vi "Load saved scan settings_arbitray cluster elements.vi"(8 "error in (no error)":errorcluster, 11 "User name":string) -> (0 "error out":errorcluster, 1 "Scan settings array":T1[](array[typedef]) {"J-t Illumination conditions" items=["Light only", "Dark only", "Light then dark", "Dark then light"]; "No. of scan rate steps" min=1.0 step=1.0; "Illumination conditions" items=["Light only", "Dark only", "Light then dark", "Dark then light", "Light then dark then light", "Dark then light then dark"]; "Time Constant (s)" items=["0.003", "0.01", "0.03", "0.1", "0.3", "1", "3", "10", "30", "100"]; "Only repeat for best pixel" items=["only for best pixel", "for best 2 pixels", "for best 3 pixels", "for best 4 pixels", "for best 5 pixels", "for best 6 pixels", "for best 7 pixels", "for all pixels"]; "No. of repeat scans" min=1.0 step=1.0; "EQE best pixel only" items=["only the best pixel", "the best 2 pixel", "the best 3 pixel", "the best 4 pixel", "the best 5 pixel", "the best 6 pixel", "the best 7 pixel", "all pixels"]; "P dep best pixel only" items=["only the best pixel", "the best 2 pixels", "the best 3 pixels", "the best 4 pixels", "the best 5 pixels", "the best 6 pixels", "the best 7 pixels", "all pixels"]; "Max power best pixel only" items=["only the best pixel", "the best 2 pixels", "the best 3 pixels", "the best 4 pixels", "the best 5 pixels", "the best 6 pixels", "the best 7 pixels", "all pixels"]; "J-t best pixel only" items=["only the best pixel", "the best 2 pixels", "the best 3 pixels", "the best 4 pixels", "the best 5 pixels", "the best 6 pixels", "the best 7 pixels", "all pixels"]; "Integration time" items=["Fast", "Normal", "High Accuracy"]; "Stabilisation mode" items=["V", "I"]; "Measurement delay (ms)" min=10.0}, 3 "Scan settings name array":string[](array[string]), 4 "Settings folder path":path)   [LabVIEW 2011]
uses:
  TypeDefs/Scan settings.ctl
  TypeDefs/Settings Boolean.ctl
  <vilib>/Utility/file.llb/Write To Spreadsheet File (string).vi
  <vilib>/Utility/file.llb/Read From Spreadsheet File (string).vi
panel:
  in  "Deafult_std":string[](array[string])=["1", "0", "-1.4", "0.1", "0.02", "10", "1", "0", "5", "0", "-1.4", "0", "0", "0", "0", "1", "1", "0", "0", "1", "0", "1", "0.7", "60", "0", "7", "0", "0", "0", "0", "0", "300", "900", "5", "100", "2", "3", "90", "2", "1", "2", "1", "1", "1", "0", "1", "0", "200", "0"]
  in  "Deafult_inv":string[](array[string])=["1", "0", "-0.1", "1.4", "0.02", "10", "1", "1", "0", "0", "1.4", "0", "0", "0", "0", "1", "1", "0", "0", "1", "0", "1", "0.7", "60", "0", "7", "0", "0", "0", "0", "0", "300", "900", "5", "100", "2", "3", "90", "2", "1", "2", "1", "1", "1", "0", "1", "0", "200", "0"]
  out "String":string
  out "all rows":string[][](array[string])
  in  "Scan settings":T1={"J-V scan"=TRUE, "J-t scan"=FALSE, "Min voltage (V)"=0.0, "Max voltage (V)"=1.4, "Step (V)"=0.01, "Measurement delay (ms)"=10.0, "1st scan FB-SC"=TRUE, "Inverted structure"=FALSE, "Stabilisation time (s)"=0.0, "Stabilisation mode"=0, "Stabilisation value (V or A) "=0.0, "Step time (s)"=1.0, "Integration time"=0, "Repeat light scans"=FALSE, "Stabilisation in the dark?"=FALSE, "J-t Min (V)"=0.0, "J-t Max (V)"=1.4, "J-t Step (V)"=0.01, "Max. power stabilisation"=FALSE, "J-t 1st scan FB-SC"=TRUE, "J-t Inverted structure"=FALSE, "Max power tracking"=FALSE, "Vmp (V)"=0.7, "Total stabilisation time (s)"=100.0, "J-t best pixel only"=0, "Max power best pixel only"=0, "Vmp from J-V scan"=FALSE, "Intensity dependence"=FALSE, "P dep best pixel only"=0, "External quantum efficiency"=FALSE, "EQE best pixel only"=0, "WL min (nm)"=300.0, "WL max (nm)"=900.0, "WL step (nm)"=5.0, "Wait (ms)"=100.0, "No. of repeat scans"=2.0, "Only repeat for best pixel"=0, "Chopper Freq.  (Hz)"=90.0, "Time Constant (s)"=2.0, "Stabilisation time step (s)"=1.0, "Illumination conditions"=2, "Scan rate min (V/s)"=0.1, "Scan rate max (V/s)"=1.0, "No. of scan rate steps"=1.0, "Scan rate voltage step priority"=FALSE, "Scan rate measurement delay priority"=FALSE, "J-t Illumination conditions"=0, "White bias  (no. of suns)"=200.0, "Max P stab. Specific voltage"=FALSE} {"J-t Illumination conditions" items=["Light only", "Dark only", "Light then dark", "Dark then light"]; "No. of scan rate steps" min=1.0 step=1.0; "Illumination conditions" items=["Light only", "Dark only", "Light then dark", "Dark then light", "Light then dark then light", "Dark then light then dark"]; "Time Constant (s)" items=["0.003", "0.01", "0.03", "0.1", "0.3", "1", "3", "10", "30", "100"]; "Only repeat for best pixel" items=["only for best pixel", "for best 2 pixels", "for best 3 pixels", "for best 4 pixels", "for best 5 pixels", "for best 6 pixels", "for best 7 pixels", "for all pixels"]; "No. of repeat scans" min=1.0 step=1.0; "EQE best pixel only" items=["only the best pixel", "the best 2 pixel", "the best 3 pixel", "the best 4 pixel", "the best 5 pixel", "the best 6 pixel", "the best 7 pixel", "all pixels"]; "P dep best pixel only" items=["only the best pixel", "the best 2 pixels", "the best 3 pixels", "the best 4 pixels", "the best 5 pixels", "the best 6 pixels", "the best 7 pixels", "all pixels"]; "Max power best pixel only" items=["only the best pixel", "the best 2 pixels", "the best 3 pixels", "the best 4 pixels", "the best 5 pixels", "the best 6 pixels", "the best 7 pixels", "all pixels"]; "J-t best pixel only" items=["only the best pixel", "the best 2 pixels", "the best 3 pixels", "the best 4 pixels", "the best 5 pixels", "the best 6 pixels", "the best 7 pixels", "all pixels"]; "Integration time" items=["Fast", "Normal", "High Accuracy"]; "Stabilisation mode" items=["V", "I"]; "Measurement delay (ms)" min=10.0}
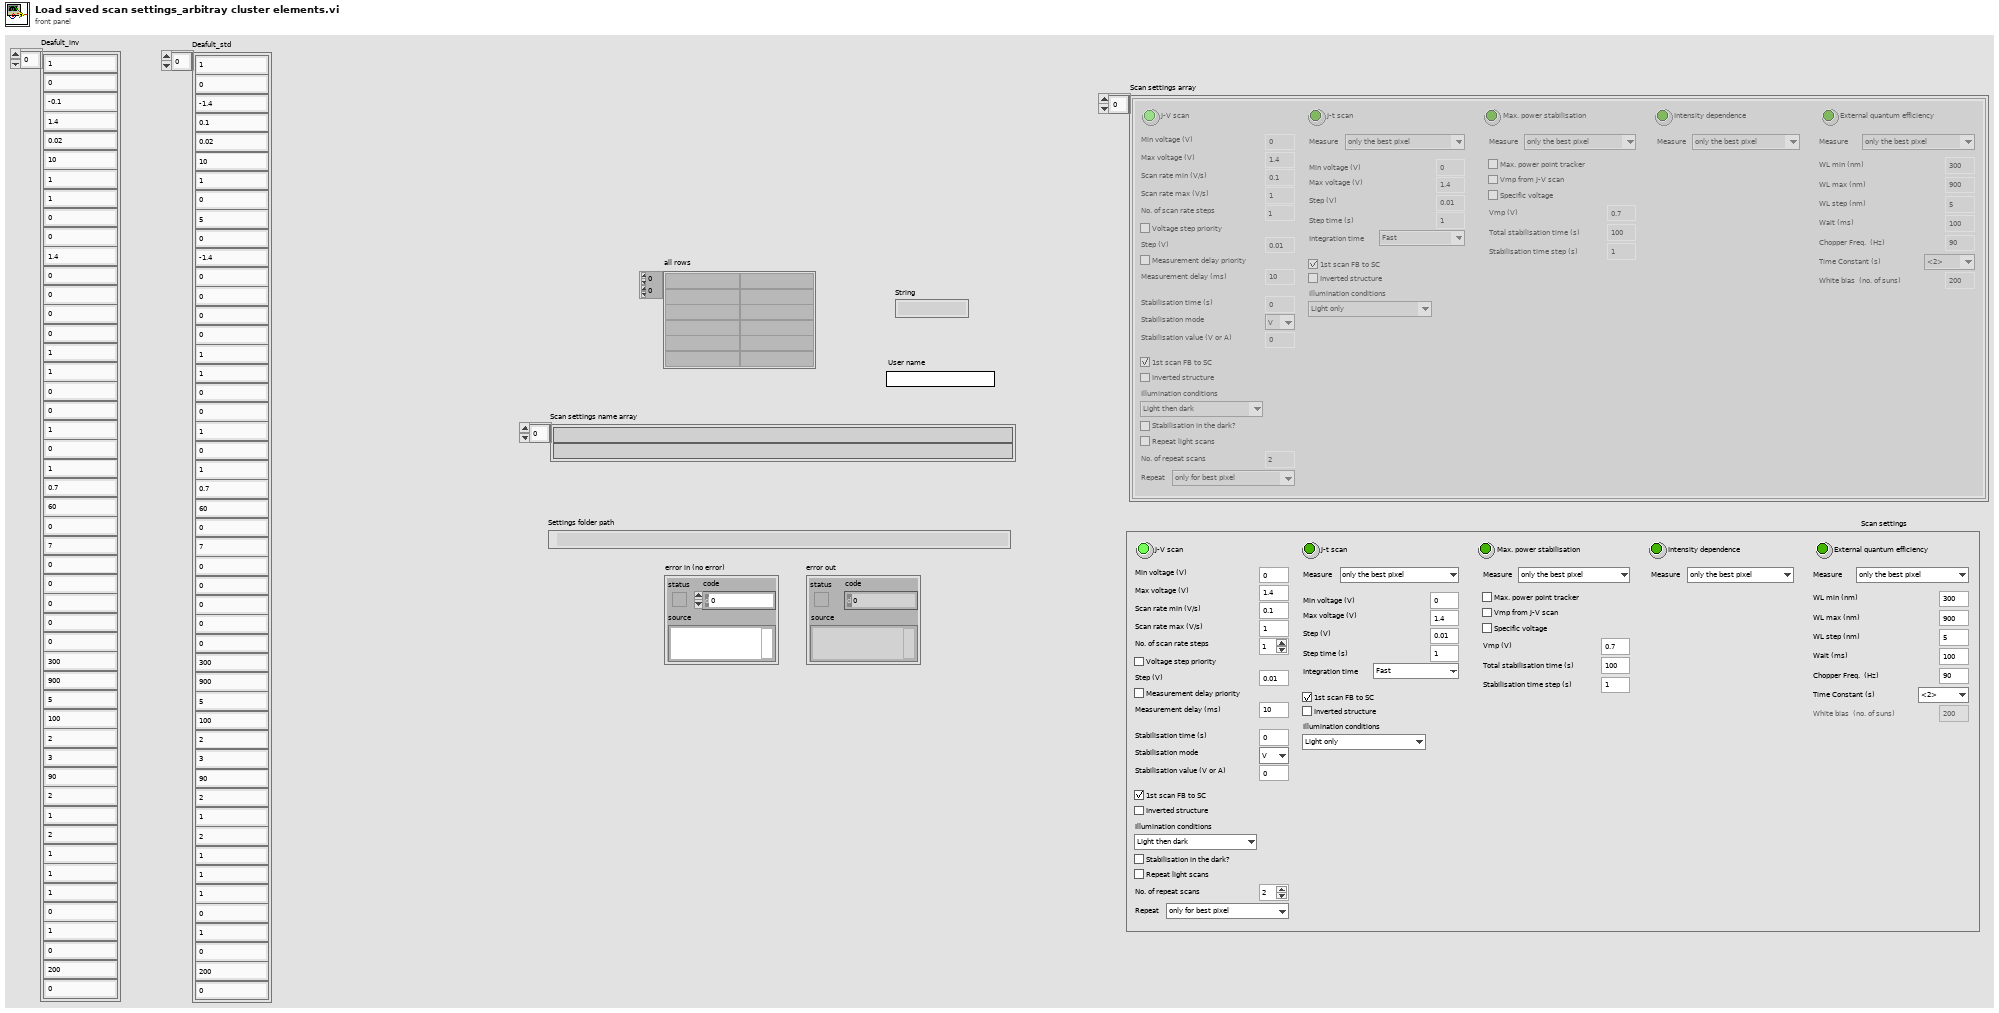
[diagram p1: front panel]
types:
  T1 = typedef "Scan settings.ctl" = cluster{"J-V scan":T2, "J-t scan":bool, "Min voltage (V)":dbl, "Max voltage (V)":dbl, "Step (V)":dbl, "Measurement delay (ms)":dbl, "1st scan FB-SC":bool, "Inverted structure":bool, "Stabilisation time (s)":dbl, "Stabilisation mode":u16, "Stabilisation value (V or A) ":dbl, "Step time (s)":dbl, "Integration time":u16, "Repeat light scans":bool, "Stabilisation in the dark?":bool, "J-t Min (V)":dbl, "J-t Max (V)":dbl, "J-t Step (V)":dbl, "Max. power stabilisation":bool, "J-t 1st scan FB-SC":bool, "J-t Inverted structure":bool, "Max power tracking":bool, "Vmp (V)":dbl, "Total stabilisation time (s)":dbl, "J-t best pixel only":u16, "Max power best pixel only":u16, "Vmp from J-V scan":bool, "Intensity dependence":bool, "P dep best pixel only":u16, "External quantum efficiency":bool, "EQE best pixel only":u16, "WL min (nm)":dbl, "WL max (nm)":dbl, "WL step (nm)":dbl, "Wait (ms)":dbl, "No. of repeat scans":dbl, "Only repeat for best pixel":u16, "Chopper Freq.  (Hz)":dbl, "Time Constant (s)":dbl, "Stabilisation time step (s)":dbl, "Illumination conditions":u16, "Scan rate min (V/s)":dbl, "Scan rate max (V/s)":dbl, "No. of scan rate steps":dbl, "Scan rate voltage step priority":bool, "Scan rate measurement delay priority":bool, "J-t Illumination conditions":u16, "White bias  (no. of suns)":dbl, "Max P stab. Specific voltage":bool}
  T2 = typedef "Settings Boolean.ctl" = bool
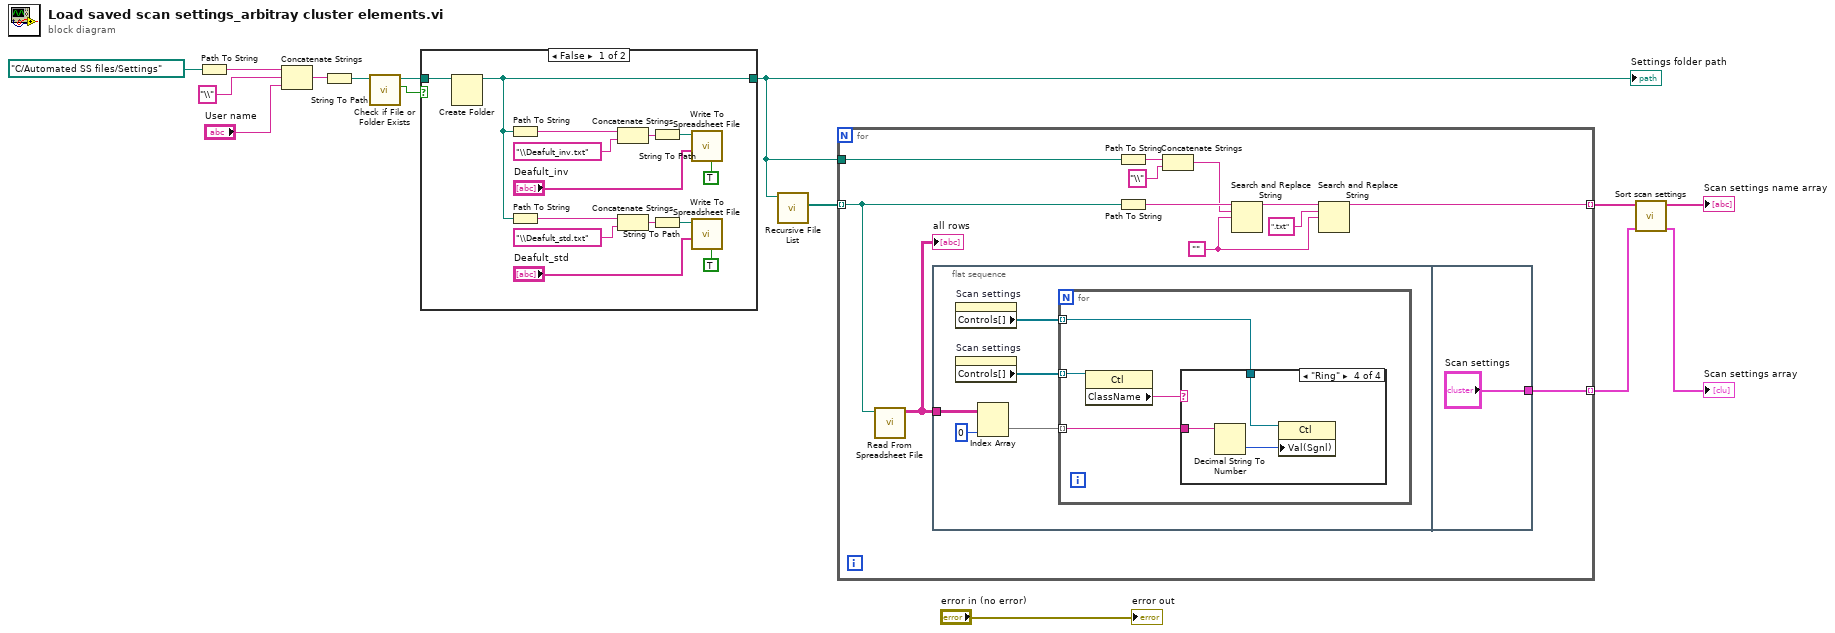
[diagram p0: block diagram]
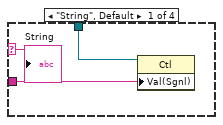
[diagram p3: hidden frame]
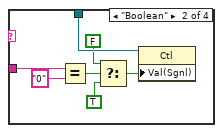
[diagram p4: hidden frame]
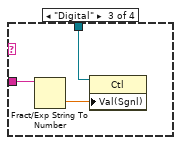
[diagram p5: hidden frame]
diagram:
  n1 = Path To String(path=path "C:/Automated SS files/Settings") -> (string=w9:string)
  n2 = Concatenate Strings(w9, "\\", "User name") -> (w1:string)
  n3 = String To Path(string=w1) -> (path=w4:path)
  n4 = call <vilib>:"Check if File or Folder Exists.vi"("path"=w4) -> ("file or folder exists?"=w6:bool, "dup path"=w5:path)  [unwired: 8 in, 1 out]
  n5 = case shown="False" w6 {
    tunnel: w5 -> [w29 w30]
    tunnel: [w21 w30] -> w2
    frame False {
      n6 = Create Folder(path (use dialog)=w29) -> (created path=w21:path)  [unwired: 2 in, 2 out]
      n7 = Path To String(path=w21) -> (string=w26:string)
      n8 = Path To String(path=w21) -> (string=w22:string)
      n9 = Concatenate Strings(w26, "\\Deafult_inv.txt") -> (w25:string)
      n10 = Concatenate Strings(w22, "\\Deafult_std.txt") -> (w19:string)
      n11 = String To Path(string=w25) -> (path=w24:path)
      n12 = String To Path(string=w19) -> (path=w20:path)
      n13 = call-poly <vilib>:"Write To Spreadsheet File.vi"("transpose? (no:F)"=TRUE, "1D data"="Deafult_inv", "file path (dialog if empty)"=w24) -> ()  [unwired: 5 in, 1 out]
      n14 = call-poly <vilib>:"Write To Spreadsheet File.vi"("transpose? (no:F)"=TRUE, "1D data"="Deafult_std", "file path (dialog if empty)"=w20) -> ()  [unwired: 5 in, 1 out]
    }
    frame True {
    }
  }
  "Settings folder path" <- w2
  n15 = call <vilib>:"Recursive File List.vi"("Folder Path"=w2) -> ("All Files in Dir"=w15:path[])  [unwired: 6 in, 4 out]
  n16 = for {
    tunnel: w15 -> [w32] mode=indexing
    tunnel: w2 -> [w34]
    tunnel: [w33] -> w13 mode=indexing
    tunnel: [w31] -> w11 mode=indexing
    w40 = ""
    n17 = call-poly <vilib>:"Read From Spreadsheet File.vi"("file path (dialog if empty)"=w32) -> ("all rows"=w35:string[][])  [unwired: 6 in, 4 out]
    "all rows" <- w35
    n18 = flat-sequence {
      tunnel: w35 -> [w45]
      tunnel: ["Scan settings"] -> w31
      frame #0 {
        n19 = property on="Scan settings" class="Clust (strict)"() -> ("Controls[]"=w46:refnum<vi>[])  [unwired: 2 in, 2 out]
        n20 = property on="Scan settings" class="Clust (strict)"() -> ("Controls[]"=w47:refnum<vi>[])  [unwired: 2 in, 2 out]
        n21 = Index Array(array=w45, index (col)=0 ("disabled index (col)")) -> (element=w43:string[])  [unwired: 1 in]
        n22 = for {
          tunnel: w47 -> [w51] mode=indexing
          tunnel: w46 -> [w49] mode=indexing
          tunnel: w43 -> [w48] mode=indexing
          n23 = property class="Ctl"(reference=w51) -> ("ClassName"=w50:string)  [unwired: 1 in, 2 out]
          n24 = case shown="\"Ring\"" w50 {
            selector: w50 -> [w52 _ _ _]
            tunnel: w49 -> [w54 w61 w64 w66]
            tunnel: w48 -> [w53 w60 w63 w67]
            frame "String", Default {
              n25 = property class="Ctl"(reference=w54, "Val(Sgnl)"=w53) -> ()  [unwired: 1 in, 2 out]
              "String" <- w52
            }
            frame "Boolean" {
              n26 = Equal?(x=w60, y="0") -> (x = y?=w58:bool)
              n27 = Select(t=FALSE, s=w58, f=TRUE) -> (s? t:f=w55:bool)
              n28 = property class="Ctl"(reference=w61, "Val(Sgnl)"=w55) -> ()  [unwired: 1 in, 2 out]
            }
            frame "Digital" {
              n29 = Fract/Exp String To Number(string=w63) -> (number=w62:dbl)  [unwired: 3 in, 1 out]
              n30 = property class="Ctl"(reference=w64, "Val(Sgnl)"=w62) -> ()  [unwired: 1 in, 2 out]
            }
            frame "Ring" {
              n31 = Decimal String To Number(string=w67) -> (number=w65:i32)  [unwired: 2 in, 1 out]
              n32 = property class="Ctl"(reference=w66, "Val(Sgnl)"=w65) -> ()  [unwired: 1 in, 2 out]
            }
          }
        }
      }
      frame #1 {
      }
    }
    n33 = Path To String(path=w34) -> (string=w38:string)
    n34 = Path To String(path=w32) -> (string=w41:string)
    n35 = Concatenate Strings(w38, "\\") -> (w36:string)
    n36 = Search and Replace String(input string=w41, search string=w36, replace string=w40) -> (result string=w39:string)  [unwired: 5 in, 3 out]
    n37 = Search and Replace String(input string=w39, search string=".txt", replace string=w40) -> (result string=w33:string)  [unwired: 5 in, 3 out]
  }
  n38 = call "Sort scan settings.vi"("Scan settings array"=w11, "Setting name array"=w13) -> ("Sorted settings array"=→"Scan settings array":T1[], "Sorted name array"=→"Scan settings name array":string[])  [unwired: 7 in]
  "error out" <- "error in (no error)"
